vi "Lab5Done.vi"() -> ()   [LabVIEW 2024]
panel:
  out "Pump":bool
  out "System":bool
  out "Height (cm)":dbl(slide) scale=0.0..60.0
  out "Low Pressure":bool
  in  "stop":bool
  out "Pressure in H2O":dbl(slide) scale=0.0..25.0
  out "Amps, mA":dbl(slide) scale=0.0..25.0
  out "AtoD Hex":i16 format="%x"
  out "AtoD":dbl
  out "SCC,V":dbl(slide) scale=0.0..7.0
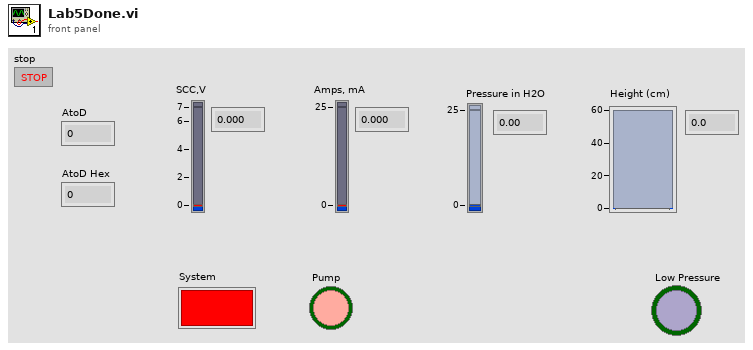
[diagram p1: front panel]
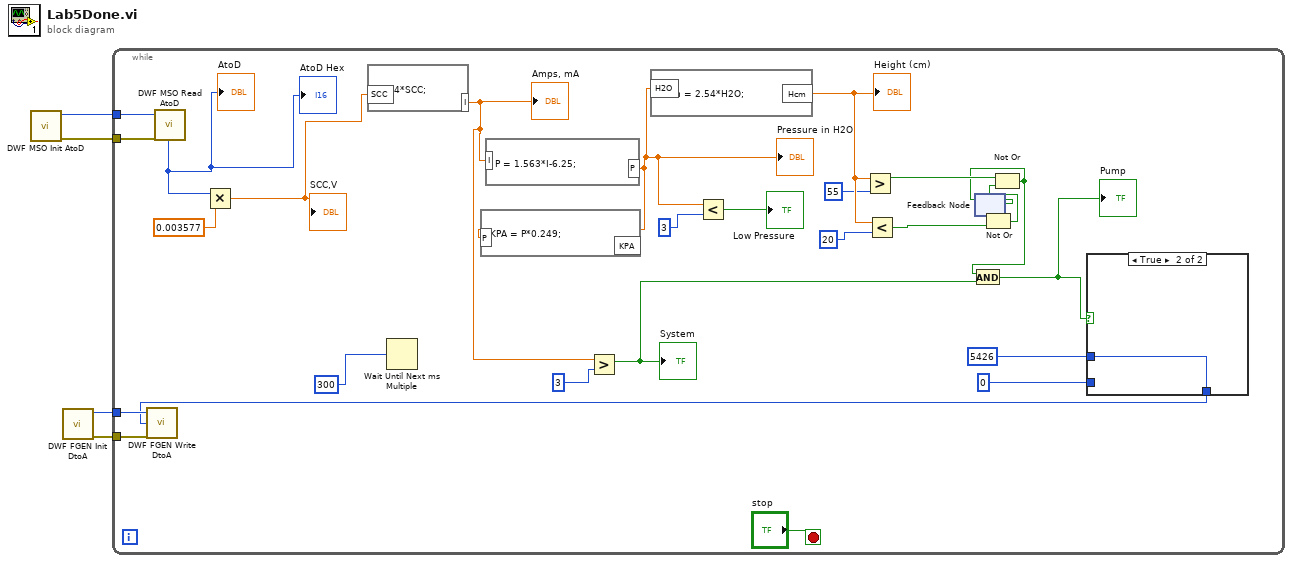
[diagram p0: block diagram]
diagram:
  n1 = call "DWF MSO Init AtoD.vi"() -> ("Error Out"=w3:errorcluster, "Instrument Handle Out"=w4:u32)  [unwired: 10 in]
  n2 = call "DWF FGEN Init DtoA.vi"() -> ("Error Out"=w1:errorcluster, "Instrument Handle Out"=w2:u32)  [unwired: 10 in]
  n3 = while {
    tunnel: w4 -> [w31]
    tunnel: w3 -> [w30]
    tunnel: w2 -> [w18]
    tunnel: w1 -> [w17]
    stop <- "stop" stop-if-true
    n4 = call "DWF MSO Read AtoD.vi"("Instrument Handle In AtoD"=w31, "Error In"=w30) -> ("AtoD"=w28:i16)  [unwired: 12 in, 1 out]
    "AtoD" <- w28
    "AtoD Hex" <- w28
    n5 = Multiply(x=w28, y=0.003577) -> (x*y=w27:dbl)
    "SCC,V" <- w27
    n6 = formula code="I = 4*SCC;"("SCC"=w27) -> ("I"=w22:dbl)
    "Amps, mA" <- w22
    n7 = Wait Until Next ms Multiple(millisecond multiple=300) -> ()  [unwired: 1 out]
    n8 = formula code="P = 1.563*I-6.25;"("I"=w22) -> ("P"=w13:dbl)
    "Pressure in H2O" <- w13
    n9 = formula code="KPA = P*0.249;"("P"=w13) -> ()  [unwired: 1 out]
    n10 = Greater?(x=w22, y=3) -> (0:w7:bool)
    "System" <- w7
    n11 = formula code="Hcm = 2.54*H2O;"("H2O"=w13) -> ("Hcm"=w11:dbl)
    "Height (cm)" <- w11
    n12 = Less?(x=w13, y=3) -> (x < y?=→"Low Pressure":bool)
    n13 = Greater?(x=w11, y=55) -> (0:w20:bool)
    n14 = Less?(x=w11, y=20) -> (x < y?=w19:bool)
    n15 = feedback #1() -> (w8:bool)  [unwired: 1 in]
    n16 = Not Or(1:w19, 2:w8) -> (0:w9:bool)
    n17 = Not Or(1:w9, 2:w20) -> (0:w6:bool)
    n18 = And(x=w6, y=w7) -> (x .and. y?=w5:bool)
    "Pump" <- w5
    n19 = feedback-in #1(w6) -> ()
    n20 = case shown="True" w5 {
      tunnel: 5426 -> [_ w33]
      tunnel: [w32 w33] -> w14
      tunnel: 0 -> [w32 _]
      frame False {
      }
      frame True {
      }
    }
    n21 = call "DWF FGEN Write DtoA.vi"("Error In"=w17, "Raw Data"=w14, "Instrument Handle In"=w18) -> ()  [unwired: 1 in, 2 out]
  }
